vi "Initialize.vi"(8 "error in (no error)":errorcluster, 9 "Ordered deps":refnum<class "ProjectItem.lvclass">[](array[class]), 11 "BuildManager in":refnum<class "BuildManager.lvclass">) -> (0 "error out":errorcluster, 3 "BuildManager out":refnum<class "BuildManager.lvclass">)   [LabVIEW 2019, in "SolutionBuilder.lvlib" / "BuildManager.lvclass"]
uses:
  BuildManager.lvclass
  ProjectItem/ProjectItem.lvclass
  BuildManager.lvclass/BuildManager.ctl
  SolutionBuilder.lvlib
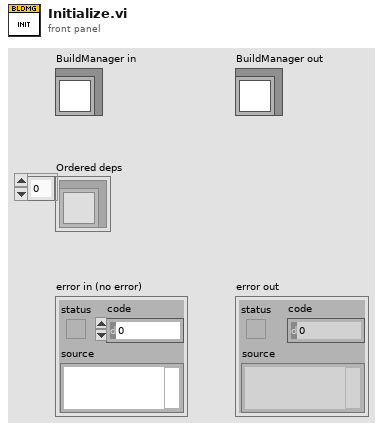
[diagram p1: front panel]
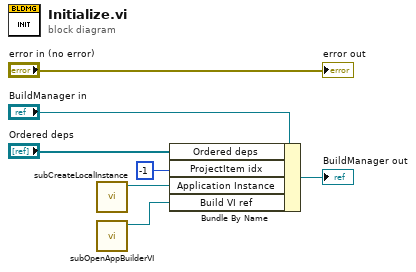
[diagram p0: block diagram]
diagram:
  n1 = call "subCreateLocalInstance.vi"() -> ("Application out"=w1:refnum<vi>)  [unwired: 11 in]
  n2 = call "subOpenAppBuilderVI.vi"() -> ("VI ref"=w2:refnum<vi>)  [unwired: 10 in, 1 out]
  n3 = Bundle By Name(cluster="BuildManager in", "Ordered deps"="Ordered deps", "ProjectItem idx"=-1, "Application Instance"=w1, "Build VI ref"=w2) -> (→"BuildManager out":refnum<class "BuildManager.lvclass">)
  "error out" <- "error in (no error)"
